vi "write_settings_file.vi"(8 "error in (no error)":errorcluster, 11 "GenericPlugin in":refnum<class "GenericComponent.lvclass">) -> (0 "error out":errorcluster, 1 "settings name (wihout \".xml\" file ending)":string, 2 "cancelled?":bool, 3 "GenericPlugin out":refnum<class "GenericComponent.lvclass">)   [LabVIEW 2010, in "GenericComponent.lvclass"]
uses:
  GenericComponent.lvclass
  <vilib>/regexp/Match Regular Expression.xnode
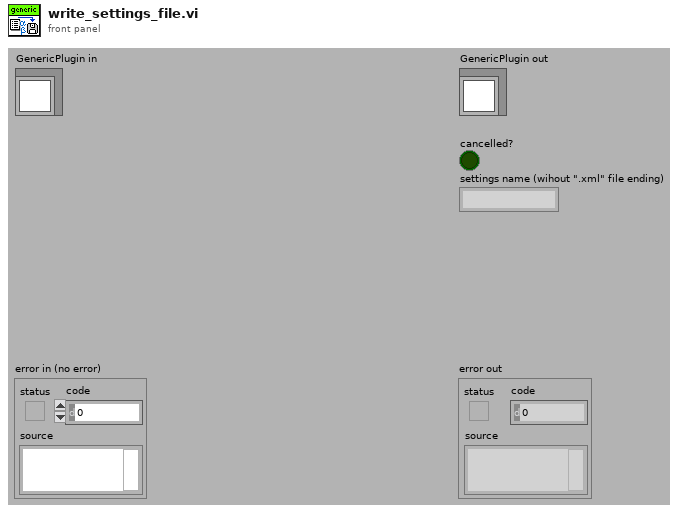
[diagram p1: front panel]
types:
  T1 = enum16{"open", "replace", "create", "open or create", "replace or create", "replace or create with confirmation"}
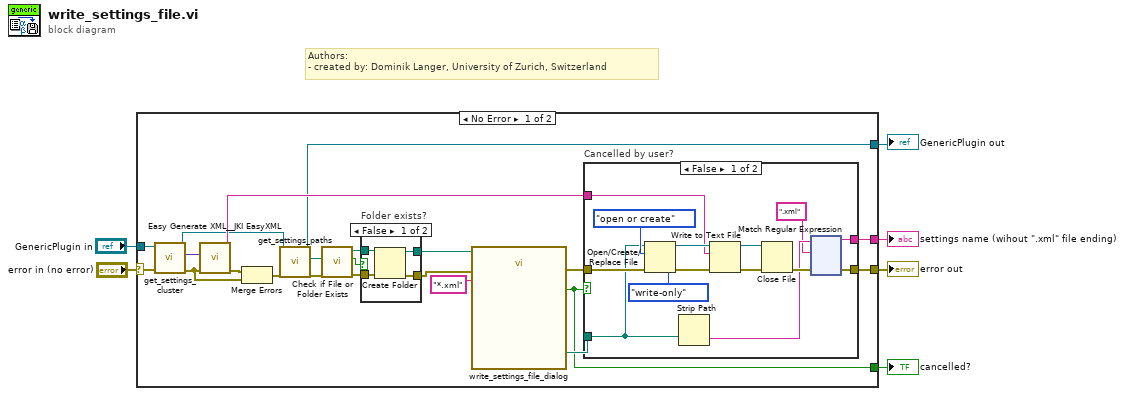
[diagram p0: block diagram]
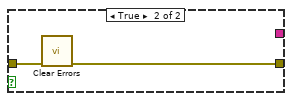
[diagram p3: hidden frame]
diagram:
  # "Authors: \n- created by: Dominik Langer, University of Zurich, Switzerland"
  n1 = case shown="No Error" "error in (no error)" {
    selector: "error in (no error)" -> [w23 w163]
    tunnel: [w24 w163] -> w5
    tunnel: [w19 w162] -> w3
    tunnel: "GenericPlugin in" -> [w21 w162]
    tunnel: [w8 _] -> w2
    tunnel: [w7 _] -> w1
    frame No Error {
      n2 = call-dynamic "get_settings_cluster.vi"("error in (no error)"=w23, "GenericPlugin in"=w21) -> ("error out"=w16:errorcluster, "settings cluster"=w22:variant, "GenericPlugin out"=w20:refnum<class "GenericComponent.lvclass">)  [unwired: 7 in]
      n3 = call <vilib>:"Easy Generate XML__JKI EasyXML.vi"("error in (no error)"=w16, "LabVIEW Data"=w22) -> ("error out"=w18:errorcluster, "XML String"=w28:string)  [unwired: 8 out]
      n4 = Merge Errors(w18, w16) -> (w17:errorcluster)
      n5 = call-dynamic "get_settings_paths.vi"("error in (no error)"=w17, "GenericComponent in"=w20) -> ("error out"=w13:errorcluster, "settings folder for a specific component"=w14:path, "GenericComponent out"=w19:refnum<class "GenericComponent.lvclass">)  [unwired: 4 in, 3 out]
      n6 = call <vilib>:"Check if File or Folder Exists.vi"("error in (no error)"=w13, "path"=w14) -> ("error out"=w11:errorcluster, "file or folder exists?"=w10:bool, "dup path"=w12:path)  [unwired: 7 in]
      n7 = case "Folder exists?" shown="False" w10 {
        tunnel: [w32 w34] -> w15
        tunnel: w12 -> [w31 w33]
        tunnel: w11 -> [w30 w34]
        tunnel: [w29 w33] -> w9
        frame False {
          n8 = Create Folder(path (use dialog)=w31, error in=w30) -> (created path=w29:path, error out=w32:errorcluster)  [unwired: 1 in, 1 out]
        }
        frame True {
        }
      }
      n9 = call "write_settings_file_dialog.vi"("start path"=w9, "error in"=w15, "pattern (all files)"="*.xml") -> ("selected path"=w25:path, "cancelled"=w8:bool, "error out"=w26:errorcluster)  [unwired: 9 in, 1 out]
      n10 = case "Cancelled by user?" shown="False" w8 {
        tunnel: w28 -> [w46 _]
        tunnel: w26 -> [w41 w161]
        tunnel: w25 -> [w40 _]
        tunnel: [w38 w160] -> w24
        tunnel: [w36 _] -> w7
        frame False {
          n11 = Open/Create/Replace File(file path (use dialog)=w40, error in=w41, operation (0:open)=T1."open or create", access (0:read/write)=enum16{"read/write", "read-only", "write-only"}."write-only") -> (refnum out=w47:refnum<file>, error out=w48:errorcluster)  [unwired: 3 out]
          n12 = Strip Path(path=w40) -> (name=w37:string)  [unwired: 1 out]
          n13 = Write to Text File(file (use dialog)=w47, text=w46, error in=w48) -> (refnum out=w44:refnum<file>, error out=w45:errorcluster)  [unwired: 2 out]
          n14 = Close File(refnum=w44, error in=w45) -> (error out=w39:errorcluster)  [unwired: 1 out]
          n15 = xnode "Match Regular Expression"("input string"=w37, "regular expression"=".xml", "error in"=w39) -> ("before match"=w36:string, "error out"=w38:errorcluster)  [unwired: 3 in, 3 out]
        }
        frame True {
          n16 = call <vilib>:"Clear Errors.vi"("error in (no error)"=w161) -> ("error out"=w160:errorcluster)  [unwired: 6 in]
        }
      }
    }
    frame Error {
    }
  }
  "error out" <- w5
  "GenericPlugin out" <- w3
  "cancelled?" <- w2
  "settings name (wihout \".xml\" file ending)" <- w1
